vi "Page_Windows_Security_Quit.vi"(6 "output cluster":T1, 8 "error in (no error)":errorcluster, 9 "data":variant, 10 "Target":refnum<vi>, 11 "AB_Application in":refnum<class "AB_Application.lvclass">) -> (0 "error out":errorcluster, 3 "AB_Application out":refnum<class "AB_Application.lvclass">)   [LabVIEW 2020, in "AB_Application.lvclass"]
uses:
  <vilib>/AppBuilder/AB_Classes/Application/AB_Application.lvclass
  <vilib>/AppBuilder/AB_Classes/Application/AB_Application.lvclass/AB_Application.ctl
  <resource>/Framework/Providers/Common/provcom_BrowseProjectFile.ctl
  <resource>/Framework/Providers/Builds/AppBuilder/AB_UI_Page_Windows_Security_References.ctl
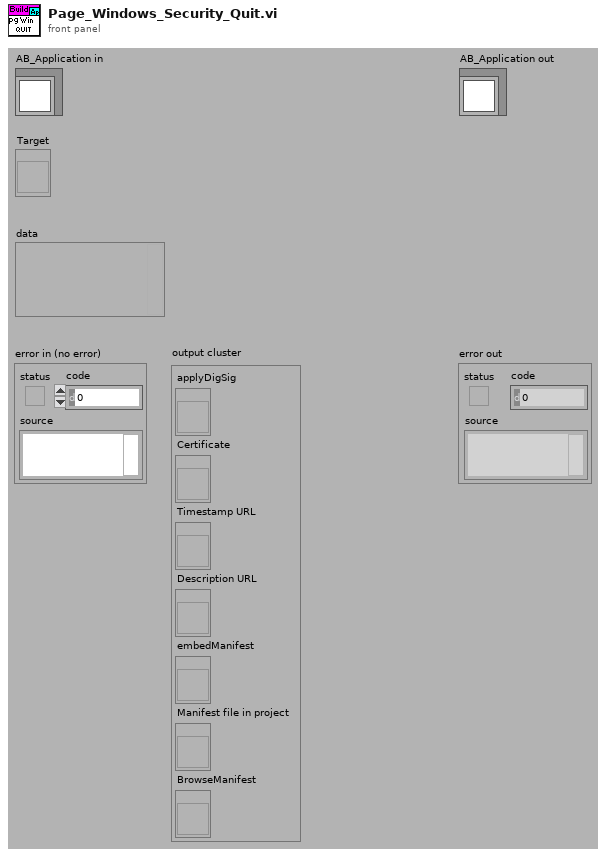
[diagram p1: front panel]
types:
  T1 = typedef "AB_UI_Page_Windows_Security_References.ctl" = cluster{"applyDigSig":refnum<vi>, "Certificate":refnum<vi>, "Timestamp URL":refnum<vi>, "Description URL":refnum<vi>, "embedManifest":refnum<vi>, "Manifest file in project":refnum<vi>, "BrowseManifest":refnum<vi>}
  T2 = typedef "AB_Application.ctl" = cluster{"INI_path":path, "INI_itemID":string, "INI_GUID":string, "aliasPath":path, "aliasItemID":string, "aliasGUID":string, "waitDebugging":bool, "copyErrors":bool, "useFFRTE":bool, "includeHWConfig":bool, "showHWConfig":bool, "winsec.certificate":string, "winsec.timestamp":string, "winsec.description":string, "winsec.manifestItemID":string, "winsec.manifestPath":path, "web service itemIDs":string[], "Embedded Server Configuration":T3, "Server Type":enum32{"NI Web Server", "Application Web Server"}}
  T3 = typedef "AB_Embedded_Server_Configuration.ctl" = cluster{"HTTP enabled?":bool, "HTTP port":i32, "HTTPS enabled?":bool, "HTTPS port":i32, "SSL certificate file":path}
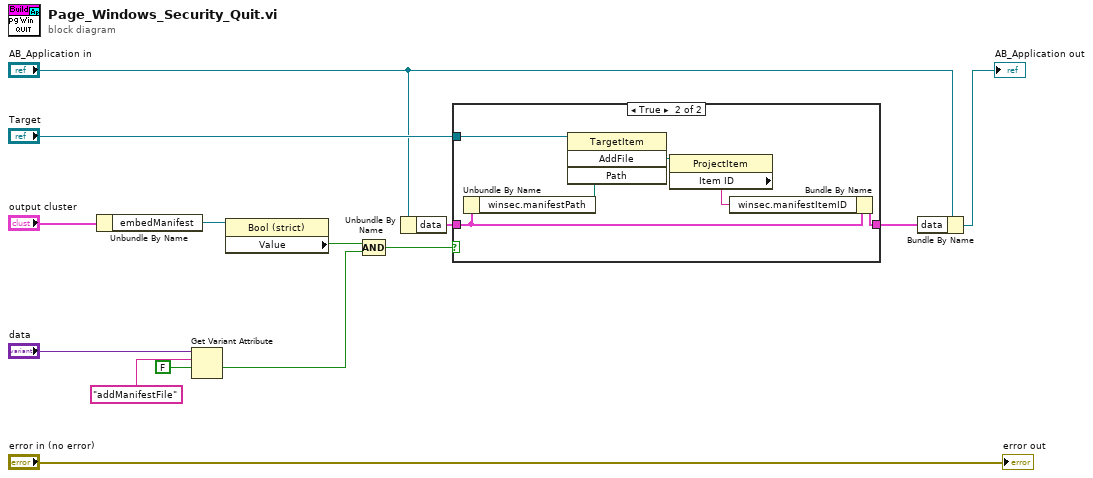
[diagram p0: block diagram]
diagram:
  n1 = Unbundle By Name("output cluster") -> ("embedManifest"=w9:refnum<vi>)
  n2 = Get Variant Attribute(Variant="data", name="addManifestFile", default value (empty Variant)=FALSE) -> (value=w7:bool)  [unwired: 1 in, 3 out]
  n3 = property class="Bool (strict)"(reference=w9) -> ("Value"=w8:bool)  [unwired: 1 in, 2 out]
  n4 = Compound Arithmetic op=AND(w8, w7) -> (w5:bool)
  n5 = Unbundle By Name("AB_Application in") -> ("data"=w4:T2)
  n6 = case shown="True" w5 {
    tunnel: "Target" -> [_ w20]
    tunnel: w4 -> [w15 w18]
    tunnel: [w15 w16] -> w1
    frame False {
    }
    frame True {
      n7 = Unbundle By Name(w18) -> ("winsec.manifestPath"=w19:path)
      n8 = invoke class="TargetItem" method="AddFile"(reference=w20, "Path"=w19) -> ("AddFile"=w21:refnum<vi>)  [unwired: 2 in, 3 out]
      n9 = property class="ProjectItem"(reference=w21) -> ("Item ID"=w17:string)  [unwired: 1 in, 2 out]
      n10 = Bundle By Name(cluster=w18, "winsec.manifestItemID"=w17) -> (w16:T2)
    }
  }
  n11 = Bundle By Name(cluster="AB_Application in", "data"=w1) -> (→"AB_Application out":refnum<class "AB_Application.lvclass">)
  "error out" <- "error in (no error)"
